vi "sim_stage_test.vi"() -> ()   [LabVIEW 2024]
uses:
  O:/DSG/Tyler/EIC/DIRC/daq/automated/Thorlabs.MotionControl.Controls.dll
  Thorlabs.MotionControl.Controls.dll
  O:/DSG/Tyler/EIC/DIRC/daq/automated/Thorlabs.MotionControl.DeviceManagerCLI.dll
  Thorlabs.MotionControl.DeviceManagerCLI.dll
panel:
  in  "Control2":refnum<k24>(container)
  out "error out":errorcluster
  in  "stop":bool
  in  "Control":refnum<k24>(container)
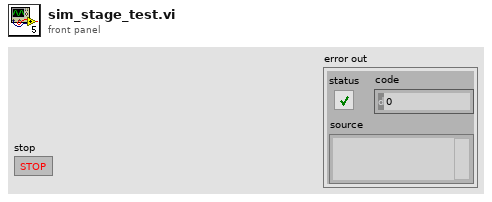
[diagram p1: front panel]
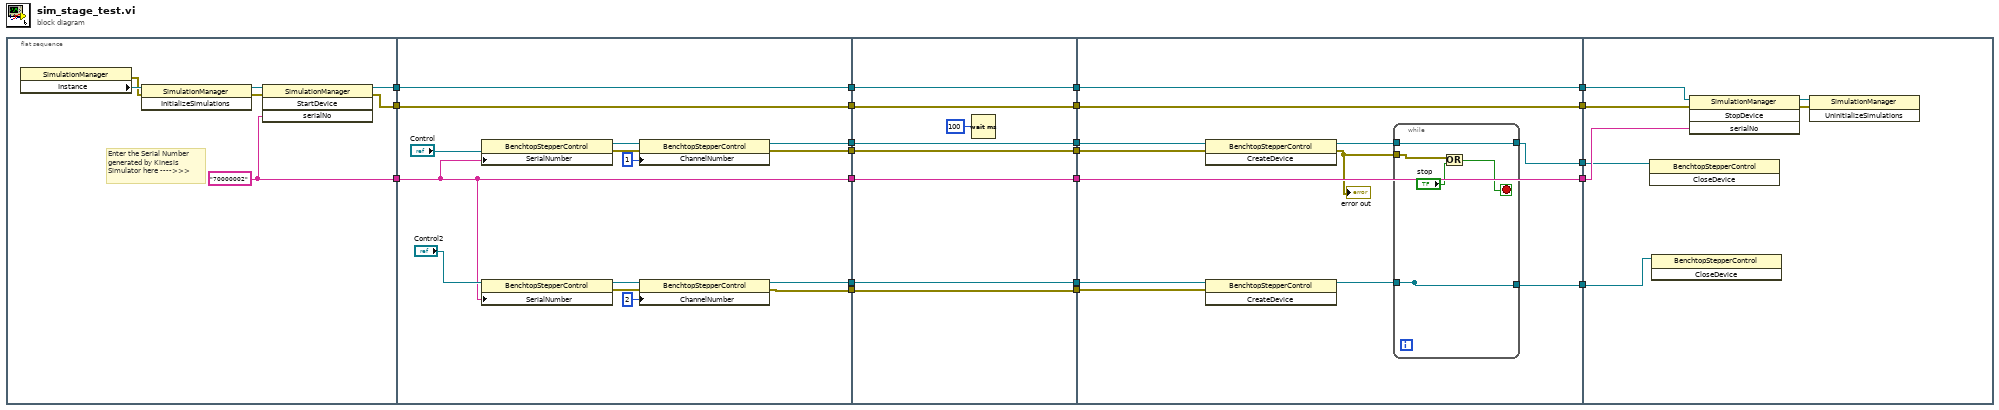
[diagram p0: block diagram]
diagram:
  n1 = flat-sequence {
    tunnel: [w27] -> w18
    tunnel: [w26] -> w17
    tunnel: [w23] -> w16
    tunnel: w18 -> [w32]
    tunnel: [w32] -> w15
    tunnel: w17 -> [w44]
    tunnel: [w44] -> w13
    tunnel: w16 -> [w43]
    tunnel: [w43] -> w11
    tunnel: [w40] -> w9
    tunnel: [w38] -> w7
    tunnel: [w31] -> w5
    tunnel: [w30] -> w2
    tunnel: w15 -> [w52]
    tunnel: [w52] -> w14
    tunnel: w13 -> [w51]
    tunnel: [w51] -> w12
    tunnel: w11 -> [w50]
    tunnel: [w50] -> w10
    tunnel: w9 -> [w49]
    tunnel: [w49] -> w8
    tunnel: w7 -> [w48]
    tunnel: [w48] -> w6
    tunnel: w5 -> [w46]
    tunnel: [w46] -> w4
    tunnel: [w45] -> w3
    tunnel: w2 -> [w45]
    tunnel: w14 -> [w62]
    tunnel: [w62] -> w22
    tunnel: [w63] -> w21
    tunnel: w12 -> [w63]
    tunnel: [w64] -> w20
    tunnel: w10 -> [w64]
    tunnel: [w60] -> w19
    tunnel: w8 -> [w58]
    tunnel: w6 -> [w57]
    tunnel: w4 -> [w56]
    tunnel: w3 -> [w55]
    tunnel: [w53] -> w1
    tunnel: w22 -> [w75]
    tunnel: w21 -> [w74]
    tunnel: w20 -> [w73]
    tunnel: w19 -> [w71]
    tunnel: w1 -> [w70]
    frame #0 {
      w27 = "70000002" ("serialNo")
      # "Enter the Serial Number\ngenerated by Kinesis \nSimulator here ---->>>"
      n2 = property class="SimulationManager"() -> (error out=w25:errorcluster, "Instance"=w29:refnum<k24>)  [unwired: 2 in, 1 out]
      n3 = invoke class="SimulationManager" method="InitializeSimulations"(reference=w29, error in=w25) -> (reference out=w28:refnum<k24>, error out=w24:errorcluster)  [unwired: 1 in, 1 out]
      n4 = invoke class="SimulationManager" method="StartDevice"(reference=w28, error in=w24, "serialNo"=w27) -> (reference out=w26:refnum<k24>, error out=w23:errorcluster)  [unwired: 1 in, 2 out]
    }
    frame #1 {
      n5 = property class="BenchtopStepperControl"(reference="Control", "SerialNumber"=w32) -> (reference out=w41:refnum<k24>, error out=w39:errorcluster)  [unwired: 1 in]
      n6 = property class="BenchtopStepperControl"(reference="Control2", "SerialNumber"=w32) -> (reference out=w34:refnum<k24>, error out=w35:errorcluster)  [unwired: 1 in]
      n7 = property class="BenchtopStepperControl"(reference=w41, error in=w39, "ChannelNumber"=1) -> (reference out=w40:refnum<k24>, error out=w38:errorcluster)
      n8 = property class="BenchtopStepperControl"(reference=w34, error in=w35, "ChannelNumber"=2) -> (reference out=w31:refnum<k24>, error out=w30:errorcluster)
    }
    frame #2 {
      n9 = Wait (ms)(milliseconds to wait=u32 100) -> ()  [unwired: 1 out]
    }
    frame #3 {
      n10 = invoke class="BenchtopStepperControl" method="CreateDevice"(reference=w58, error in=w57) -> (reference out=w61:refnum<k24>, error out=w59:errorcluster)  [unwired: 1 in, 1 out]
      "error out" <- w59
      n11 = invoke class="BenchtopStepperControl" method="CreateDevice"(reference=w56, error in=w55) -> (reference out=w54:refnum<k24>)  [unwired: 1 in, 2 out]
      n12 = while {
        tunnel: w61 -> [w69]
        tunnel: [w69] -> w60
        tunnel: w59 -> [w68]
        tunnel: [w65] -> _
        tunnel: w54 -> [w65]
        tunnel: [w65] -> w53
        stop <- w66 stop-if-true
        n13 = Or(x=w68, y="stop") -> (x .or. y?=w66:bool)
      }
    }
    frame #4 {
      n14 = invoke class="BenchtopStepperControl" method="CloseDevice"(reference=w71) -> ()  [unwired: 2 in, 3 out]
      n15 = invoke class="BenchtopStepperControl" method="CloseDevice"(reference=w70) -> ()  [unwired: 2 in, 3 out]
      n16 = invoke class="SimulationManager" method="StopDevice"(reference=w74, error in=w73, "serialNo"=w75) -> (reference out=w76:refnum<k24>, error out=w72:errorcluster)  [unwired: 1 in, 2 out]
      n17 = invoke class="SimulationManager" method="UninitializeSimulations"(reference=w76, error in=w72) -> ()  [unwired: 1 in, 3 out]
    }
  }
